vi "Calculate Message Class Path.vi"(10 "Method VI Name":string, 11 "Actor Class Path":path) -> (2 "Message Class Path":path)   [LabVIEW 2020, in "Message Maker.lvlib"]
uses:
  Message Maker.lvlib
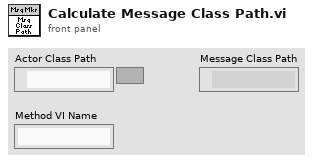
[diagram p1: front panel]
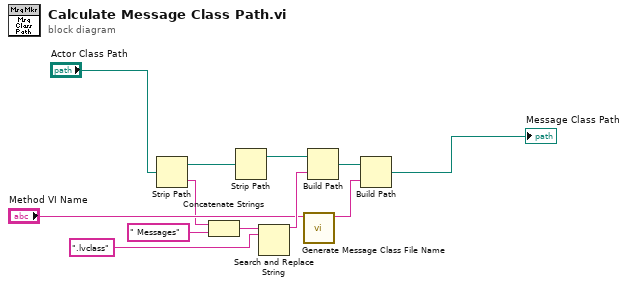
[diagram p0: block diagram]
diagram:
  n1 = Strip Path(path="Actor Class Path") -> (stripped path=w2:path, name=w7:string)
  n2 = Concatenate Strings(w7, " Messages" ("string")) -> (w10:string)
  n3 = Strip Path(path=w2) -> (stripped path=w6:path)  [unwired: 1 out]
  n4 = Search and Replace String(input string=w10, search string=".lvclass" ("string")) -> (result string=w11:string)  [unwired: 6 in, 3 out]
  n5 = call "Generate Message Class File Name.vi"("Target Method"="Method VI Name") -> ("Msg Class File Name"=w4:string)  [unwired: 10 in]
  n6 = Build Path(base path=w6, name or relative path=w11) -> (appended path=w5:path)
  n7 = Build Path(base path=w5, name or relative path=w4) -> (appended path=→"Message Class Path":path)
